vi "DiscArchiver.change file prefix.vi"(0 "i ref in":refnum<vi>, 2 "file prefix":string, 3 "ms timeout (10000)":i32=10000, 5 "error in (no error)":errorcluster) -> (14 "i ref out":refnum<vi>, 17 "timed out":bool, 19 "error out":errorcluster)   [LabVIEW 2014, in "DiscArchiver.lvlib"]
doc: "Changes the file prefix. The change becomes effective the next time a new file is opened."
uses:
  DiscArchiver.lvlib
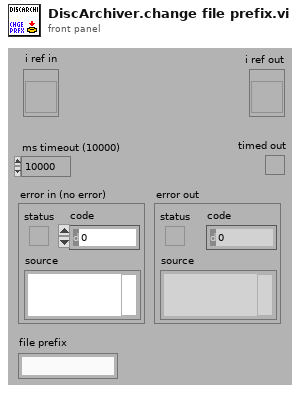
[diagram p1: front panel]
types:
  T1 = typedef "DiscArchiver.lvlib/DiscArchiver.i attribute.ctl" = cluster{"file prefix":string, "actual file":string, "nOfEvents":i32, "file":refnum<file>, "eventBuilder":string, "disc size alarm":bool, "dataDescription":string, "dataDescriptionURL":string, "eventDataURL":string, "headerID":dbl, "completeData":bool, "nOfEventsID":i32, "dataFileID":i32}
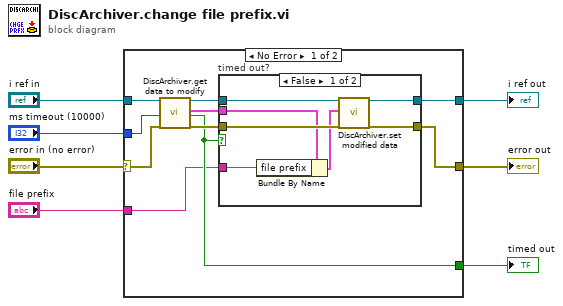
[diagram p0: block diagram]
diagram:
  n1 = case shown="No Error" "error in (no error)" {
    selector: "error in (no error)" -> [w8 w27]
    tunnel: "i ref in" -> [w17 w28]
    tunnel: [w16 w27] -> w6
    tunnel: [w15 w28] -> w5
    tunnel: "ms timeout (10000)" -> [w11 _]
    tunnel: [w10 _] -> w3
    tunnel: "file prefix" -> [w9 _]
    frame No Error {
      n2 = call "DiscArchiver.get data to modify.vi"("i ref in"=w17, "ms timeout (10000)"=w11, "error in (no error)"=w8) -> ("i ref out"=w14:refnum<vi>, "i attribute"=w12:T1, "timed out"=w10:bool, "error out"=w13:errorcluster)  [unwired: 13 in]
      n3 = case "timed out?" shown="False" w10 {
        tunnel: [w24 w25] -> w16
        tunnel: [w23 w26] -> w15
        tunnel: w14 -> [w22 w26]
        tunnel: w13 -> [w21 w25]
        tunnel: w12 -> [w19 _]
        tunnel: w9 -> [w18 _]
        frame False {
          n4 = Bundle By Name(cluster=w19, "file prefix"=w18) -> (w20:T1)
          n5 = call "DiscArchiver.set modified data.vi"("i ref in"=w22, "i attribute"=w20, "error in (no error)"=w21) -> ("i ref out"=w23:refnum<vi>, "error out"=w24:errorcluster)  [unwired: 15 in]
        }
        frame True {
        }
      }
    }
    frame Error {
    }
  }
  "error out" <- w6
  "i ref out" <- w5
  "timed out" <- w3
